vi "Scanned Write - Module.vi"(6 "Channel Type":T2, 7 "error in (no error)":errorcluster, 9 "data in":dbl[](array[numeric]), 10 "IOV ref in":T1) -> (0 "error out":errorcluster, 3 "IOV ref out":T1)   [LabVIEW 2016, in "Scan Engine Custom Device.lvlib"]
uses:
  Scan Engine Custom Device.lvlib
  Modules.lvlibp/RSI Module/Channel Type.ctl
  Type Defs/Open Module IOVs.ctl
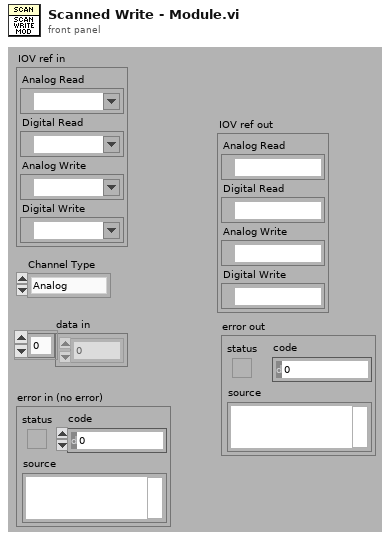
[diagram p1: front panel]
types:
  T1 = typedef "Scan Engine Custom Device.lvlib/Open Module IOVs.ctl" = cluster{"Analog Read":refnum<k21>, "Digital Read":refnum<k21>, "Analog Write":refnum<k21>, "Digital Write":refnum<k21>}
  T2 = typedef "Modules.lvlibp/RSI Module.lvclass/Channel Type.ctl" = enum16{"Analog", "Digital"}
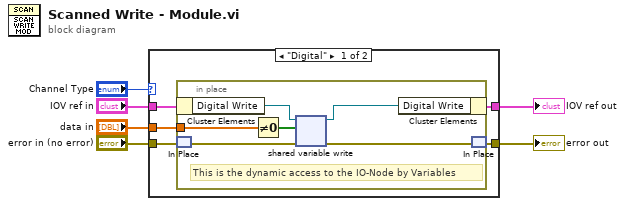
[diagram p0: block diagram]
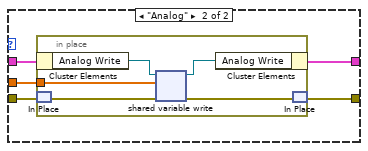
[diagram p2: hidden frame]
diagram:
  n1 = case shown="\"Digital\"" "Channel Type" {
    tunnel: "IOV ref in" -> [w10 w21]
    tunnel: "error in (no error)" -> [w7 w19]
    tunnel: [w8 w18] -> w6
    tunnel: "data in" -> [w11 w22]
    tunnel: [w9 w20] -> w1
    frame "Digital" {
      n2 = in-place {
        in-place-border: w11 -> [w17]
        # "This is the dynamic access to the IO-Node by Variables"
        n3 = in-place-cluster #1(w10) -> ("Digital Write"=w15:refnum<k21>)
        n4 = in-place-match #2(w7) -> (w12:errorcluster)
        n5 = Not Equal To 0?(x=w17) -> (x != 0?=w16:bool[])
        n6 = shared-variable-write(w15, w12, w16) -> (w14:refnum<k21>, w13:errorcluster)
        n7 = in-place-cluster #1("Digital Write"=w14) -> (w9:T1)
        n8 = in-place-match #2(w13) -> (w8:errorcluster)
      }
    }
    frame "Analog" {
      n9 = in-place {
        in-place-border: w22 -> [w25]
        n10 = in-place-cluster #3(w21) -> ("Analog Write"=w27:refnum<k21>)
        n11 = in-place-match #4(w19) -> (w24:errorcluster)
        n12 = shared-variable-write(w27, w24, w25) -> (w26:refnum<k21>, w23:errorcluster)
        n13 = in-place-cluster #3("Analog Write"=w26) -> (w20:T1)
        n14 = in-place-match #4(w23) -> (w18:errorcluster)
      }
    }
  }
  "error out" <- w6
  "IOV ref out" <- w1
